vi "Decorator3_Main.vi"() -> (0 "error out":errorcluster)   [LabVIEW 2020]
uses:
  EncryptionDecorator_class/EncryptionDecorator.lvclass
  C:/Projects/DesignPatterns/Decorator3/DataSource_interface/DataSource.lvclass
  FileDataSource_class/FileDataSource.lvclass
  CompressionDecorator_class/CompressionDecorator.lvclass
  DataSource_interface/DataSource.lvclass
panel:
  in  "Add Compression Decorator":bool
  in  "Add Encryption Decorator":bool
  out "resulting string":string
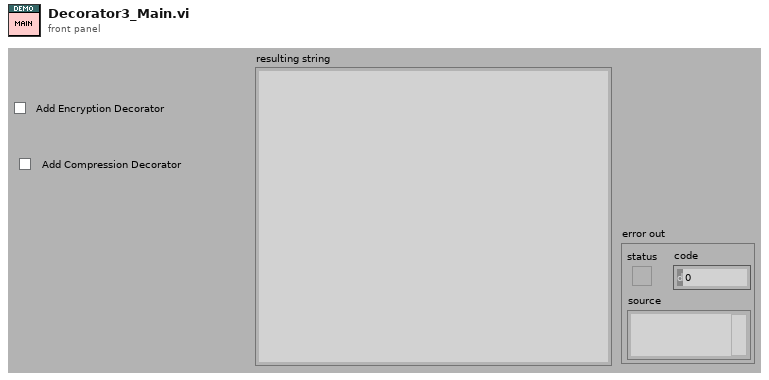
[diagram p1: front panel]
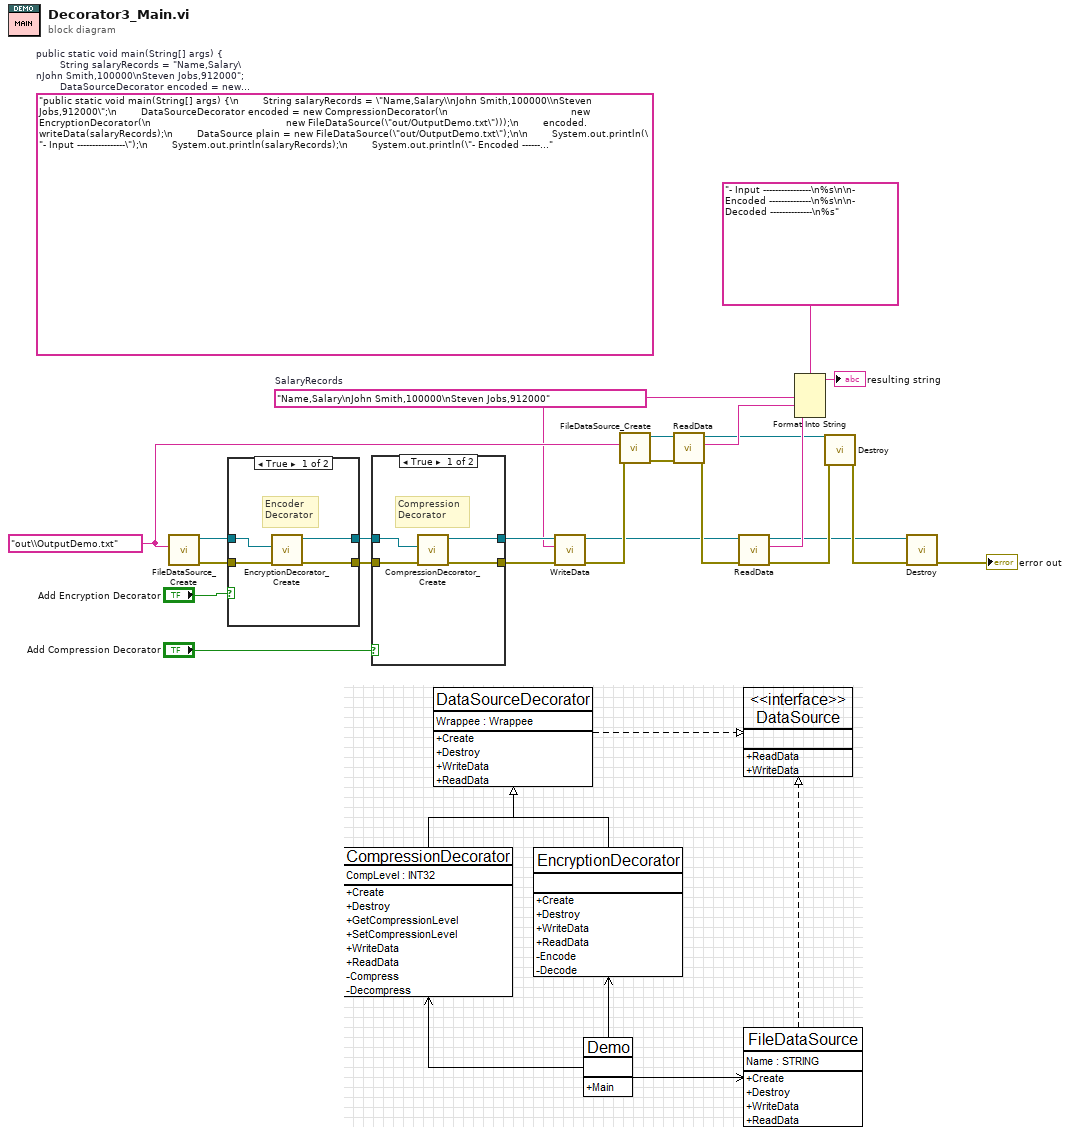
[diagram p0: block diagram]
diagram:
  w19 = "out\\OutputDemo.txt" ("Name")
  w5 = "Name,Salary\nJohn Smith,100000\nSteven Jobs,912000"  # SalaryRecords
  (unwired) "public static void main(String[] args) {\n        String salaryRecords = \"Name,Salary\\nJohn Smith,100000\\nSteven Jobs,912000\";\n        DataSourceDecorator encoded = new CompressionDecorator(\n                                         new EncryptionDecorator(\n                                             new FileDataSource(\"out/OutputDemo.txt\")));\n        encoded.writeData(salaryRecords);\n        DataSource plain = new FileDataSource(\"out/OutputDemo.txt\");\n\n        System.out.println(\"- Input ----------------\");\n        System.out.println(salaryRecords);\n        System.out.println(\"- Encoded --------------\");\n        System.out.println(plain.readData());\n        System.out.println(\"- Decoded --------------\");\n        System.out.println(encoded.readData());\n    }"  # public static void main(String[] args) {         String salaryRecords = "Name,Salary\nJohn Smith,100000\nSteven Jobs,912000";         DataSourceDecorator encoded = new CompressionDecorator(                                          new EncryptionDecorator(                                              new FileDataSource("out/OutputDemo.txt")));         encoded.writeData(salaryRecords);         DataSource plain = new FileDataSource("out/OutputDemo.txt");          System.out.println("- Input ----------------");         System.out.println(salaryRecords);         System.out.println("- Encoded --------------");         System.out.println(plain.readData());         System.out.println("- Decoded --------------");         System.out.println(encoded.readData());     }
  n1 = call "FileDataSource_Create.vi"("Name"=w19) -> ("error out"=w22:errorcluster, "reference out"=w3:refnum<class "FileDataSource.lvclass">)  [unwired: 9 in]
  n2 = case shown="True" "Add Encryption Decorator" {
    tunnel: [w28 w29] -> w23
    tunnel: w22 -> [w27 w30]
    tunnel: [w26 w30] -> w21
    tunnel: w3 -> [w25 w29]
    frame True {
      # "Encoder\nDecorator"
      n3 = call "EncryptionDecorator_Create.vi"("error in (no error)"=w27, "Source"=w25) -> ("error out"=w26:errorcluster, "reference out"=w28:refnum<class "EncryptionDecorator.lvclass">)  [unwired: 8 in]
    }
    frame False {
    }
  }
  n4 = case shown="True" "Add Compression Decorator" {
    tunnel: w23 -> [w34 w35]
    tunnel: w21 -> [w33 w36]
    tunnel: [w32 w36] -> w9
    tunnel: [w31 w35] -> w8
    frame True {
      # "Compression\nDecorator"
      n5 = call "CompressionDecorator_Create.vi"("error in (no error)"=w33, "Source"=w34) -> ("error out"=w32:errorcluster, "reference out"=w31:refnum<class "CompressionDecorator.lvclass">)  [unwired: 8 in]
    }
    frame False {
    }
  }
  n6 = call-dynamic "WriteData.vi"("Error In"=w9, "Data"=w5, "object in"=w8) -> ("Error Out"=w7:errorcluster, "object out"=w6:refnum<class "DataSource.lvclass">)  [unwired: 7 in]
  n7 = call "FileDataSource_Create.vi"("error in (no error)"=w7, "Name"=w19) -> ("error out"=w18:errorcluster, "reference out"=w17:refnum<class "FileDataSource.lvclass">)  [unwired: 8 in]
  n8 = call-dynamic "ReadData.vi"("Error In"=w18, "reference in"=w17) -> ("Error Out"=w15:errorcluster, "Return(STRING)"=w16:string, "reference out"=w13:refnum<class "FileDataSource.lvclass">)  [unwired: 7 in]
  n9 = call-dynamic "ReadData.vi"("Error In"=w15, "object in"=w6) -> ("Error Out"=w12:errorcluster, "Return(STRING)"=w14:string, "object out"=w10:refnum<class "DataSource.lvclass">)  [unwired: 7 in]
  n10 = Format Into String(format string="- Input ----------------\n%s\n\n- Encoded --------------\n%s\n\n- Decoded --------------\n%s", w5, w16, w14) -> (resulting string=→"resulting string":string)  [unwired: 2 in, 1 out]
  n11 = call-dynamic "Destroy.vi"("error in (no error)"=w12, "reference in"=w13) -> ("error out"=w11:errorcluster)  [unwired: 8 in, 1 out]
  n12 = call-dynamic "Destroy.vi"("Error In"=w11, "object in"=w10) -> ("Error Out"=→"error out":errorcluster)  [unwired: 8 in, 1 out]
